vi "xy图.vi"() -> ()   [LabVIEW 2018]
panel:
  out "XY图 3":cluster{dbl, dbl, dbl}[](graph)
  out "XY图 2":cluster{dbl[], dbl[]}(graph)
  out "XY图":cluster{"X":dbl, "Y":dbl}[](graph)
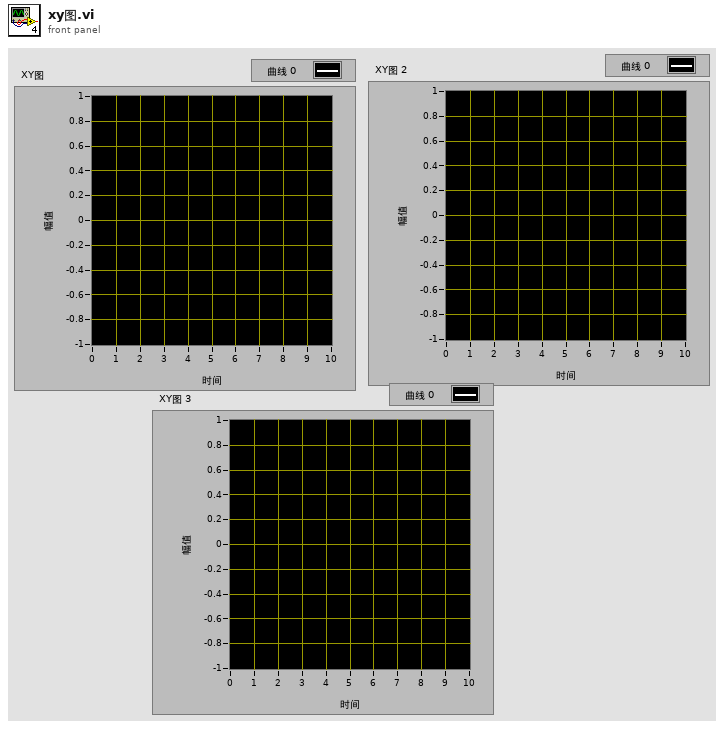
[diagram p1: front panel]
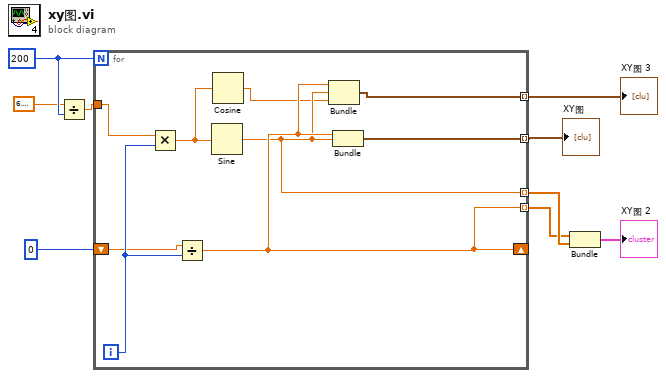
[diagram p0: block diagram]
diagram:
  w9 = 200
  n1 = Divide(x=6.283185307179586, y=w9) -> (x/y=w7:dbl)
  n2 = for {
    N: w9 -> [_]
    tunnel: w7 -> [w18]
    shift-right: [w13] -> _
    shift-left: 0 -> [w15]
    tunnel: [w16] -> w5 mode=indexing
    tunnel: [w13] -> w3 mode=indexing
    tunnel: [w12] -> w4 mode=indexing
    tunnel: [w10] -> w1 mode=indexing
    i -> [w17]
    n3 = Multiply(x=w18, y=w17) -> (x*y=w14:dbl)
    n4 = Divide(x=w15, y=w17) -> (x/y=w13:dbl)
    n5 = Sine(x=w14) -> (sin(x)=w12:dbl)
    n6 = Cosine(x=w14) -> (cos(x)=w11:dbl)
    n7 = Bundle(w13, w12, w11) -> (w10:cluster{dbl, dbl, dbl})  [unwired: 1 in]
    n8 = Bundle(w13, w12) -> (w16:cluster{dbl, dbl})  [unwired: 1 in]
  }
  "XY图" <- w5
  "XY图 3" <- w1
  n9 = Bundle(w3, w4) -> (→"XY图 2":cluster{dbl[], dbl[]})  [unwired: 1 in]
